vi "Fill Function (SubVI).vi"(0 "Signals IN":T2={"Dispense"=FALSE, "Fill"=FALSE, "Spray"=FALSE, "Drain"=TRUE, "Complete"=FALSE, "Fill Error"=FALSE, "Dispense Error"=FALSE, "Fill Timeout"=FALSE, "Dispense Timeout"=FALSE}, 1 "Values IN":T3 {"Drain Time (s)" format="%.2f"; "Drain Rate (g/sec)" format="%.2f"}, 2 "FILL Setpoint (g)":dbl, 3 "Measured Mass (g)":dbl(knob) scale=0.0..1000.0, 4 "Settings":T1={"ON Settings"={"Enable Dynamic Setpoint?"=TRUE, "Enable Dynamic Dispense Time?"=TRUE, "Enable Drain Rate Functions"=TRUE, "Dispense Sample Time (s)"=0.5, "Dispense Slope Ave"=0, "ON Timeout (sec)"=600.0, "1st Setpoint (% of Target)"=0.0, "2nd Setpoint (% of Target)"=0.0, "3rd Setpoint (% of Target)"=0.0, "Measure Dispense Delay (sec)"=0.0, "Settle Slope Sample Time (s)"=0.0}, "OFF Settings"={"Drain Sample Time (s)"=0.5, "Drain Rate Ave Size"=5, "Drain Rate Limits (± g/sec)"=10.0, "Level Slope Range (± g/sec)"=0.25, "OFF Timeout (sec)"=0.0, "Near SP Slope Level (± g/sec)"=0.01, "Near Setpoint Threshold (%)"=95.0}, "Overshoot Settings"={"Time Limit (s)"=60.0, "Container MAX (g)"=1500.0, "Max FILL Slope (+/- g/sec)"=10.0, "% Overshot to Enable (>)"=0.25}, "FILL Timeout (s)"=300.0, "Full Settle Time (s)"=20.0, "Pre-Hydrate \nSpray Time (s)"=10.0, "Pre-Hydrate \nWait Time (s)"=30.0}, 9 "Main Case Change?":bool) -> (14 "Signals OUT":T2={"Dispense"=FALSE, "Fill"=FALSE, "Spray"=FALSE, "Drain"=TRUE, "Complete"=FALSE, "Fill Error"=FALSE, "Dispense Error"=FALSE, "Fill Timeout"=FALSE, "Dispense Timeout"=FALSE}, 15 "Values OUT":T3 {"Drain Time (s)" format="%.2f"; "Drain Rate (g/sec)" format="%.2f"}, 19 "Fill FN Complete":bool)   [LabVIEW 2012]
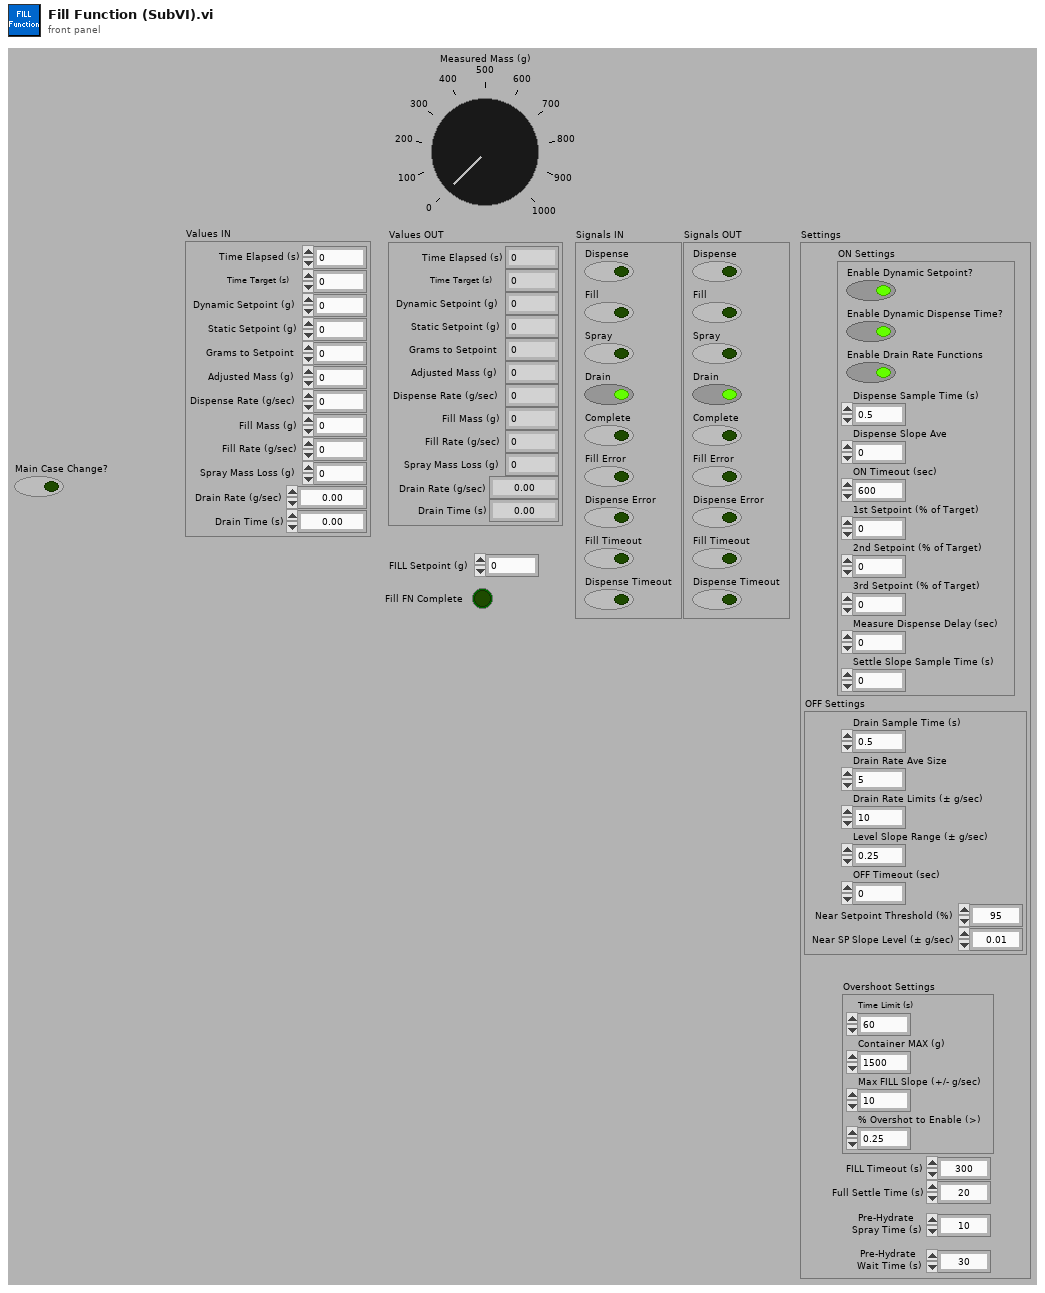
[diagram p1: front panel]
types:
  T1 = cluster{"ON Settings":cluster{"Enable Dynamic Setpoint?":bool, "Enable Dynamic Dispense Time?":bool, "Enable Drain Rate Functions":bool, "Dispense Sample Time (s)":dbl, "Dispense Slope Ave":i32, "ON Timeout (sec)":dbl, "1st Setpoint (% of Target)":dbl, "2nd Setpoint (% of Target)":dbl, "3rd Setpoint (% of Target)":dbl, "Measure Dispense Delay (sec)":dbl, "Settle Slope Sample Time (s)":dbl}, "OFF Settings":cluster{"Drain Sample Time (s)":dbl, "Drain Rate Ave Size":i32, "Drain Rate Limits (± g/sec)":dbl, "Level Slope Range (± g/sec)":dbl, "OFF Timeout (sec)":dbl, "Near SP Slope Level (± g/sec)":dbl, "Near Setpoint Threshold (%)":dbl}, "Overshoot Settings":cluster{"Time Limit (s)":dbl, "Container MAX (g)":dbl, "Max FILL Slope (+/- g/sec)":dbl, "% Overshot to Enable (>)":dbl}, "FILL Timeout (s)":dbl, "Full Settle Time (s)":dbl, "Pre-Hydrate \nSpray Time (s)":dbl, "Pre-Hydrate \nWait Time (s)":dbl}
  T2 = cluster{"Dispense":bool, "Fill":bool, "Spray":bool, "Drain":bool, "Complete":bool, "Fill Error":bool, "Dispense Error":bool, "Fill Timeout":bool, "Dispense Timeout":bool}
  T3 = cluster{"Time Elapsed (s)":dbl, "Time Target (s)":dbl, "Dynamic Setpoint (g)":dbl, "Static Setpoint (g)":dbl, "Grams to Setpoint":dbl, "Adjusted Mass (g)":dbl, "Dispense Rate (g/sec)":dbl, "Fill Mass (g)":dbl, "Fill Rate (g/sec)":dbl, "Spray Mass Loss (g)":dbl, "Drain Rate (g/sec)":dbl, "Drain Time (s)":dbl}
  T4 = enum16{"FILL INITIAL", "FILL ACTIVE", "POST FILL WAIT", "HYDRATION SPRAY", "POST HYDRATE WAIT", "FILL COMPLETE"}
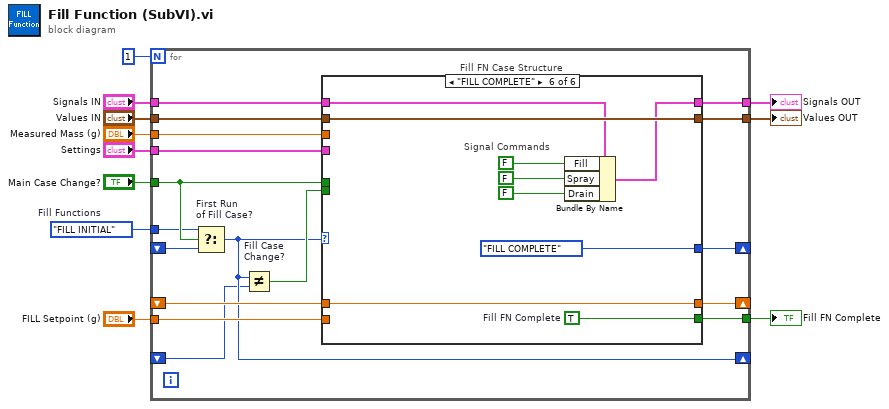
[diagram p0: block diagram]
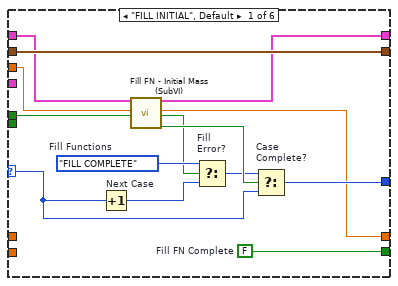
[diagram p2: hidden frame]
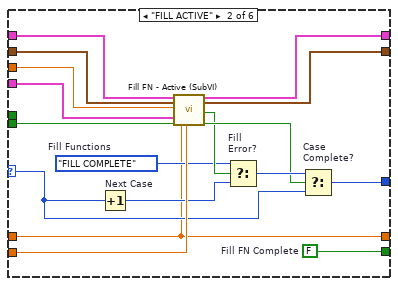
[diagram p3: hidden frame]
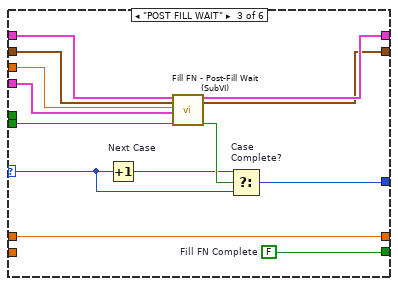
[diagram p4: hidden frame]
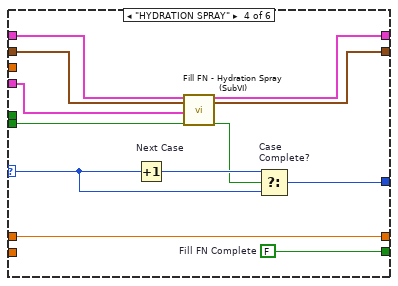
[diagram p5: hidden frame]
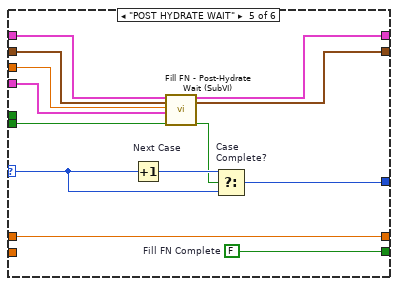
[diagram p6: hidden frame]
diagram:
  w1 = T4."FILL INITIAL"  # Fill Functions
  n1 = for {
    N: 1 -> [_]
    shift-right: [w27] -> _
    shift-left: _ -> [w28]
    tunnel: "Main Case Change?" -> [w26]
    shift-right: [w14] -> _
    shift-left: _ -> [w13]
    shift-right: [w16] -> _
    shift-left: _ -> [w20]
    tunnel: "Measured Mass (g)" -> [w24]
    tunnel: "Signals IN" -> [w23]
    tunnel: [w22] -> w7
    tunnel: "Settings" -> [w21]
    tunnel: "FILL Setpoint (g)" -> [w19]
    tunnel: "Values IN" -> [w18]
    tunnel: [w17] -> w8
    tunnel: [w15] -> w4
    tunnel: w1 -> [w12]
    n2 = Select "First Run\nof Fill Case?"(t=w12, s=w26, f=w28) -> (s? t:f=w14:T4)
    n3 = Not Equal? "Fill Case\nChange?"(x=w14, y=w13) -> (x != y?=w25:bool)
    n4 = case "Fill FN Case Structure" shown="\"FILL COMPLETE\"" w14 {
      selector: w14 -> [w38 w45 w67 w76 w91 _]
      tunnel: [w37 w56 w68 w77 w89 T4."FILL COMPLETE" ("Fill Functions")] -> w27
      tunnel: w26 -> [w30 _ _ _ _ _]
      tunnel: w25 -> [_ w55 w69 w80 w93 _]
      tunnel: w24 -> [w29 w51 w70 _ w87 _]
      tunnel: w23 -> [w32 w53 w72 w84 w97 w99]
      tunnel: [w31 w49 w71 w83 w96 w98] -> w22
      tunnel: w21 -> [_ w59 w64 w79 w86 _]
      tunnel: [w35 w48 w65 w81 w95 w106] -> w17
      tunnel: w20 -> [_ w43 w60 w73 w85 w103]
      tunnel: w19 -> [_ w52 _ _ _ _]
      tunnel: w18 -> [w35 w50 w66 w82 w94 w106]
      tunnel: [w33 w43 w60 w73 w85 w103] -> w16
      tunnel: [w34 w54 w61 w74 w88 w105] -> w15
      frame "FILL INITIAL", Default {
        w34 = FALSE  # Fill FN Complete
        w42 = T4."FILL COMPLETE"  # Fill Functions
        n5 = Increment "Next Case"(x=w38) -> (x+1=w41:T4)
        n6 = call "Fill FN - Initial Mass (SubVI).vi"("Signals IN"=w32, "Measured Mass (g)"=w29, "Main Case Change?"=w30) -> ("Signals OUT"=w31:T2, "Initial Mass"=w33:dbl, "Fill Error"=w36:bool, "Case Complete"=w40:bool)  [unwired: 1 in, 12 out]
        n7 = Select "Fill \nError?"(t=w42, s=w36, f=w41) -> (s? t:f=w39:T4)
        n8 = Select "Case\nComplete?"(t=w39, s=w40, f=w38) -> (s? t:f=w37:T4)
      }
      frame "FILL ACTIVE" {
        w46 = T4."FILL COMPLETE"  # Fill Functions
        w54 = FALSE  # Fill FN Complete
        n9 = Increment "Next Case"(x=w45) -> (x+1=w44:T4)
        n10 = call "Fill FN - Active (SubVI).vi"("Signals IN"=w53, "Values IN"=w50, "Measured Mass (g)"=w51, "Settings"=w59, "Fill Case Change?"=w55, "Initial Mass (g)"=w43, "FILL Setpoint (g)"=w52) -> ("Signals OUT"=w49:T2, "Values OUT"=w48:T3, "Fill Timeout"=w47:bool, "Case Complete"=w57:bool)  [unwired: 1 in, 8 out]
        n11 = Select "Fill \nError?"(t=w46, s=w47, f=w44) -> (s? t:f=w58:T4)
        n12 = Select "Case\nComplete?"(t=w58, s=w57, f=w45) -> (s? t:f=w56:T4)
      }
      frame "POST FILL WAIT" {
        w61 = FALSE  # Fill FN Complete
        n13 = Increment "Next Case"(x=w67) -> (x+1=w62:T4)
        n14 = call "Fill FN - Post-Fill Wait (SubVI).vi"("Signals IN"=w72, "Values IN"=w66, "Measured Mass (g)"=w70, "Settings"=w64, "Fill Case Change?"=w69) -> ("Signals OUT"=w71:T2, "Values OUT"=w65:T3, "Case Complete"=w63:bool)  [unwired: 12 out]
        n15 = Select "Case\nComplete?"(t=w62, s=w63, f=w67) -> (s? t:f=w68:T4)
      }
      frame "HYDRATION SPRAY" {
        w74 = FALSE  # Fill FN Complete
        n16 = Increment "Next Case"(x=w76) -> (x+1=w78:T4)
        n17 = call "Fill FN - Hydration Spray (SubVI).vi"("Signals IN"=w84, "Values IN"=w82, "Settings"=w79, "Fill Case Change?"=w80) -> ("Signals OUT"=w83:T2, "Values OUT"=w81:T3, "Case Complete"=w75:bool)  [unwired: 13 out]
        n18 = Select "Case\nComplete?"(t=w78, s=w75, f=w76) -> (s? t:f=w77:T4)
      }
      frame "POST HYDRATE WAIT" {
        w88 = FALSE  # Fill FN Complete
        n19 = Increment "Next Case"(x=w91) -> (x+1=w92:T4)
        n20 = call "Fill FN - Post-Hydrate Wait (SubVI).vi"("Signals IN"=w97, "Values IN"=w94, "Measured Mass (g)"=w87, "Settings"=w86, "Fill Case Change?"=w93) -> ("Signals OUT"=w96:T2, "Values OUT"=w95:T3, "Case Complete"=w90:bool)  [unwired: 12 out]
        n21 = Select "Case\nComplete?"(t=w92, s=w90, f=w91) -> (s? t:f=w89:T4)
      }
      frame "FILL COMPLETE" {
        w105 = TRUE  # Fill FN Complete
        # "Signal Commands"
        n22 = Bundle By Name(cluster=w99, "Fill"=FALSE, "Spray"=FALSE, "Drain"=FALSE) -> (w98:T2)
      }
    }
  }
  "Fill FN Complete" <- w4
  "Values OUT" <- w8
  "Signals OUT" <- w7
